vi "add wait(SubVI).vi"(10 "字符串":string) -> (1 "ok or cancel":bool, 2 "连接的字符串":string)   [LabVIEW 2019, in "Add Seq.lvlib"]
uses:
  Add Seq.lvlib
panel:
  in  "cancel":bool
  in  "ok":bool
  in  "Delay(secs)":dbl
  in  "Chamber":bool
  in  "Position":bool
  in  "Field":bool
  in  "Temperature":bool
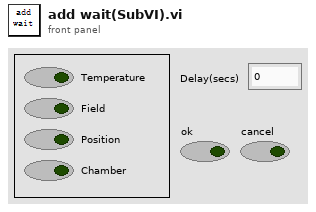
[diagram p1: front panel]
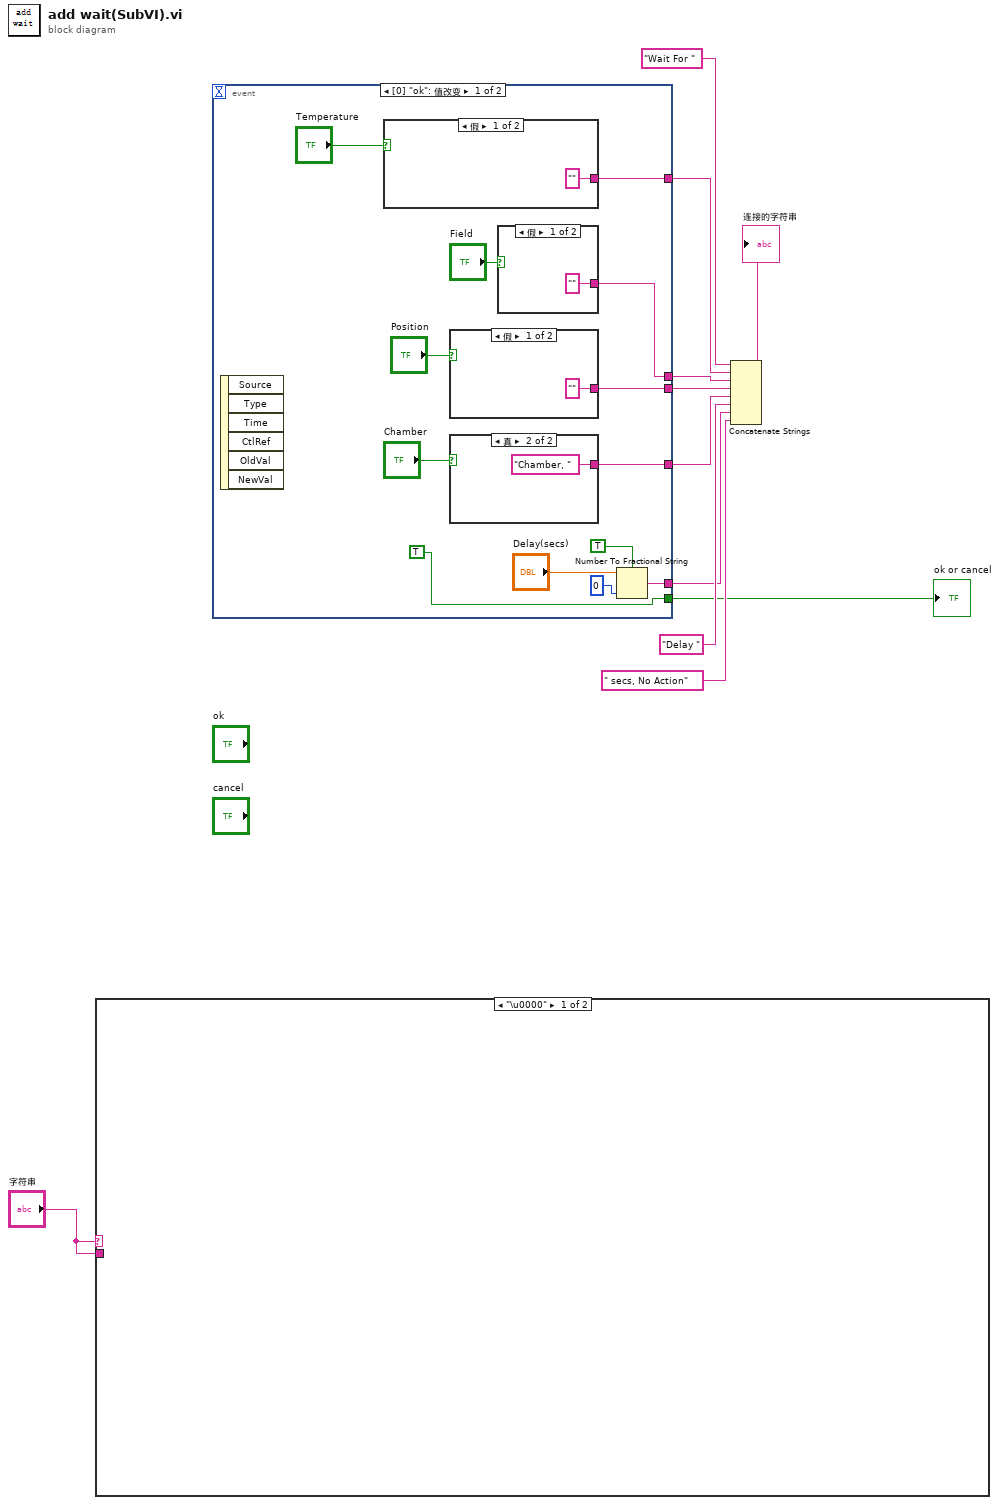
[diagram p0: block diagram]
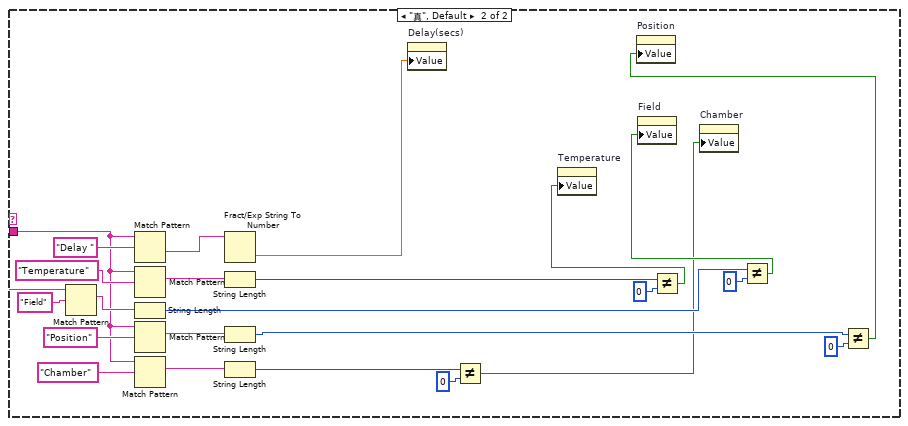
[diagram p2: hidden frame]
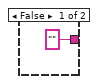
[diagram p3: hidden frame]
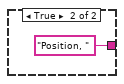
[diagram p4: hidden frame]
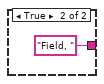
[diagram p5: hidden frame]
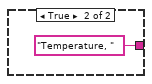
[diagram p6: hidden frame]
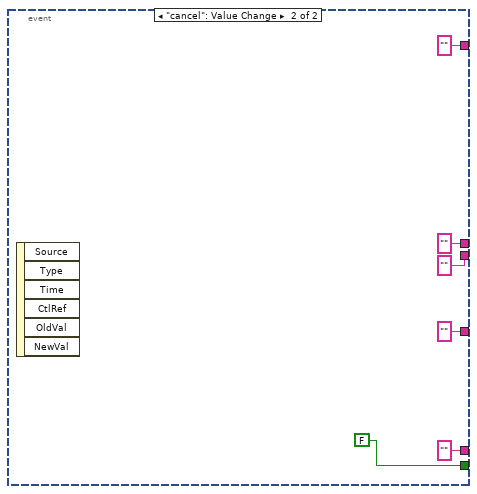
[diagram p7: hidden frame]
diagram:
  n1 = case shown="\"\"" "字符串" {
    tunnel: "字符串" -> [_ w17]
    frame "\u0000" {
    }
    frame "真", Default {
      n2 = Match Pattern(string=w17, regular expression="Field" ("正则表达式")) -> (match substring=w32:string)  [unwired: 1 in, 3 out]
      n3 = Match Pattern(string=w17, regular expression="Delay " ("正则表达式")) -> (after substring=w18:string)  [unwired: 1 in, 3 out]
      n4 = Match Pattern(string=w17, regular expression="Temperature" ("正则表达式")) -> (match substring=w35:string)  [unwired: 1 in, 3 out]
      n5 = String Length(string=w32) -> (length=w31:i32)
      n6 = Match Pattern(string=w17, regular expression="Position" ("正则表达式")) -> (match substring=w29:string)  [unwired: 1 in, 3 out]
      n7 = Match Pattern(string=w17, regular expression="Chamber" ("正则表达式")) -> (match substring=w26:string)  [unwired: 1 in, 3 out]
      n8 = Fract/Exp String To Number(string=w18) -> (number=w16:dbl)  [unwired: 3 in, 1 out]
      n9 = String Length(string=w35) -> (length=w34:i32)
      n10 = String Length(string=w29) -> (length=w28:i32)
      n11 = String Length(string=w26) -> (length=w25:i32)
      n12 = property on="Delay(secs)" class="DigNum (严格)"("Value"=w16) -> ()  [unwired: 2 in, 2 out]
      n13 = Not Equal?(x=w25, y=0) -> (x != y?=w12:bool)
      n14 = Not Equal?(x=w34, y=0) -> (x != y?=w15:bool)
      n15 = property on="Temperature" class="Bool (严格)"("Value"=w15) -> ()  [unwired: 2 in, 2 out]
      n16 = property on="Chamber" class="Bool (严格)"("Value"=w12) -> ()  [unwired: 2 in, 2 out]
      n17 = Not Equal?(x=w31, y=0) -> (x != y?=w14:bool)
      n18 = property on="Field" class="Bool (严格)"("Value"=w14) -> ()  [unwired: 2 in, 2 out]
      n19 = Not Equal?(x=w28, y=0) -> (x != y?=w13:bool)
      n20 = property on="Position" class="Bool (严格)"("Value"=w13) -> ()  [unwired: 2 in, 2 out]
    }
  }
  n21 = event shown="[0] \"ok\": 值改变" {
    selector: _ -> [_ _]
    dyn-events: _ -> [_ _]
    timeout: _ -> [_ _]
    tunnel: [w44 ""] -> w10
    tunnel: [w43 ""] -> w9
    tunnel: [w42 ""] -> w8
    tunnel: [w41 ""] -> w7
    tunnel: [w37 ""] -> w5
    tunnel: [TRUE FALSE] -> w3
    event "ok": Value Change {
      n22 = event-data() -> ()  [unwired: 1 in, 6 out]
      n23 = case shown="假" "Temperature" {
        tunnel: ["" "Temperature, "] -> w44
        frame False {
        }
        frame True {
        }
      }
      n24 = case shown="假" "Position" {
        tunnel: ["" "Position, "] -> w42
        frame False {
        }
        frame True {
        }
      }
      n25 = case shown="真" "Chamber" {
        tunnel: ["" "Chamber, "] -> w41
        frame False {
        }
        frame True {
        }
      }
      n26 = case shown="假" "Field" {
        tunnel: ["" "Field, "] -> w43
        frame False {
        }
        frame True {
        }
      }
      n27 = Number To Fractional String(use system decimal point (T)=TRUE ("使用系统小数点(T)"), number="Delay(secs)", precision (6)=i16 0 ("精度(6)")) -> (F-format string=w37:string)  [unwired: 1 in]
    }
    event "cancel": Value Change {
      n28 = event-data() -> ()  [unwired: 1 in, 6 out]
    }
  }
  "ok or cancel" <- w3
  n29 = Concatenate Strings("Wait For " ("字符串"), w10, w9, w8, w7, "Delay " ("字符串"), w5, " secs, No Action" ("字符串")) -> (→"连接的字符串":string)
